vi "Triax320 Init Wait Mess.vi"(7 "Cancelled Ref":refnum<vi>, 8 "error in (no error)":errorcluster, 9 "Stop Ref":refnum<vi>, 10 "Timeout val (ms)":dbl=100.0 min=1.0 step=1.0, 11 "Time Ref":refnum<vi>) -> (0 "error out":errorcluster, 3 "Cancelled Out":bool)   [LabVIEW 2019]
panel:
  out "Progress":u8(slide) scale=0.0..100.0
  out "Time Elapsed":dbl format="%<%M:%S>t"
  in  "stop":bool
  # "Initializing Triax 320 Spectrometer. This may take up to three minutes"
  # "Timeout"
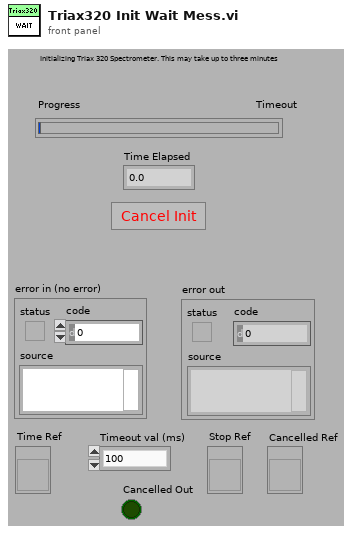
[diagram p1: front panel]
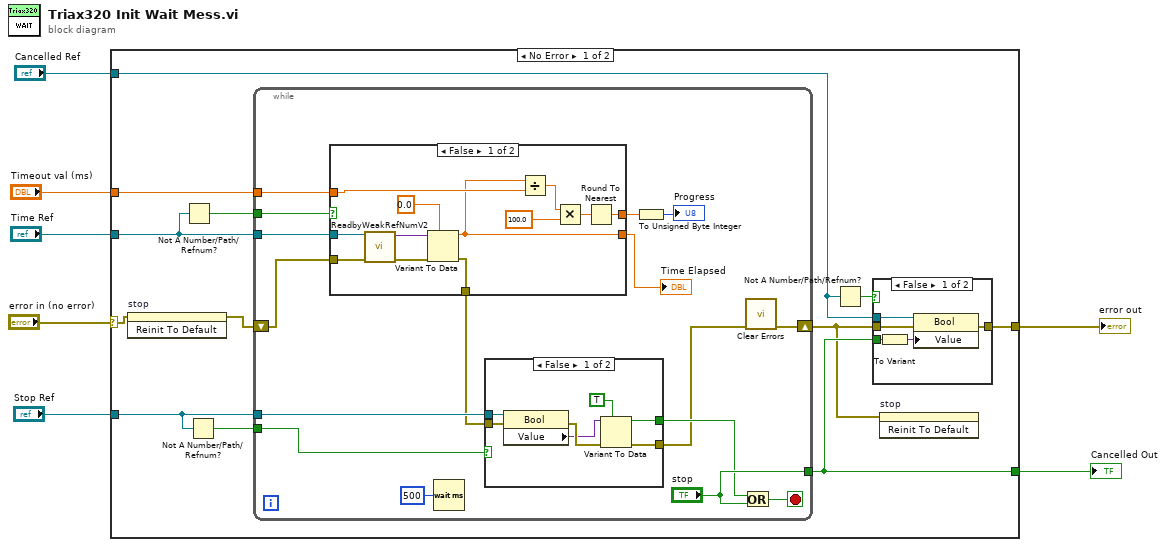
[diagram p0: block diagram]
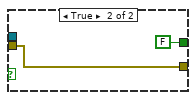
[diagram p3: hidden frame]
diagram:
  n1 = case shown="No Error" "error in (no error)" {
    selector: "error in (no error)" -> [w19 w64]
    tunnel: [w12 w64] -> w6
    tunnel: "Time Ref" -> [w17 _]
    tunnel: "Timeout val (ms)" -> [w15 _]
    tunnel: "Stop Ref" -> [w14 _]
    tunnel: [w11 _] -> w2
    tunnel: "Cancelled Ref" -> [w9 _]
    frame No Error {
      n2 = invoke on="stop" class="Bool (strict)" method="Reinit To Default"(error in=w19) -> (error out=w18:errorcluster)  [unwired: 2 in, 2 out]
      n3 = Not A Number/Path/Refnum?(number/path/refnum=w17) -> (NaN/Path/Refnum?=w16:bool)
      n4 = Not A Number/Path/Refnum?(number/path/refnum=w14) -> (NaN/Path/Refnum?=w13:bool)
      n5 = while {
        shift-right: [w26] -> w8
        shift-left: w18 -> [w38]
        tunnel: w17 -> [w39]
        tunnel: w16 -> [w37]
        tunnel: w15 -> [w36]
        tunnel: w14 -> [w31]
        tunnel: ["stop"] -> w11
        tunnel: w13 -> [w27]
        stop <- w33 stop-if-true
        n6 = case shown="False" w37 {
          tunnel: [w55 _] -> w40
          tunnel: w39 -> [w60 _]
          tunnel: w38 -> [w59 w63]
          tunnel: [w57 w63] -> w28
          tunnel: w36 -> [w56 _]
          tunnel: [w51 _] -> w35
          frame False {
            n7 = call <userlib>:"ReadbyWeakRefNumV2.vi"("error in"=w59, "Control Ref"=w60) -> ("error out"=w58:errorcluster, "Valeur"=w62:variant)  [unwired: 8 in]
            n8 = Variant To Data(error in=w58, type=0.0 ("Time Elapsed"), Variant=w62) -> (data=w55:dbl, error out=w57:errorcluster)
            n9 = Divide(x=w55, y=w56) -> (x/y=w54:dbl)
            n10 = Multiply(x=w54, y=100.0) -> (x*y=w52:dbl)
            n11 = Round To Nearest(number=w52) -> (nearest integer value=w51:dbl)
          }
          frame True {
          }
        }
        "Time Elapsed" <- w40
        n12 = Wait (ms)(milliseconds to wait=u32 500) -> ()  [unwired: 1 out]
        n13 = case shown="False" w27 {
          tunnel: w31 -> [w48 _]
          tunnel: [w44 FALSE ("stop")] -> w30
          tunnel: [w43 w50] -> w29
          tunnel: w28 -> [w42 w50]
          frame False {
            n14 = property class="Bool"(reference=w48, error in=w42) -> (error out=w47:errorcluster, "Value"=w45:variant)  [unwired: 1 out]
            n15 = Variant To Data(error in=w47, type=TRUE ("stop"), Variant=w45) -> (data=w44:bool, error out=w43:errorcluster)
          }
          frame True {
          }
        }
        n16 = To Unsigned Byte Integer(number=w35) -> (unsigned 8bit integer=→"Progress":u8)
        n17 = Or(x=w30, y="stop") -> (x .or. y?=w33:bool)
        n18 = call <vilib>:"Clear Errors.vi"("error in (no error)"=w29) -> ("error out"=w26:errorcluster)  [unwired: 5 in, 1 out]
      }
      n19 = Not A Number/Path/Refnum?(number/path/refnum=w9) -> (NaN/Path/Refnum?=w10:bool)
      n20 = case shown="False" w10 {
        tunnel: w8 -> [w24 w25]
        tunnel: [w23 w25] -> w12
        tunnel: w9 -> [w22 _]
        tunnel: w11 -> [w21 _]
        frame False {
          n21 = To Variant(anything=w21) -> (Variant=w20:variant)
          n22 = property class="Bool"(reference=w22, error in=w24, "Value"=w20) -> (error out=w23:errorcluster)  [unwired: 1 out]
        }
        frame True {
        }
      }
      n23 = invoke on="stop" class="Bool (strict)" method="Reinit To Default"(error in=w8) -> ()  [unwired: 2 in, 3 out]
    }
    frame Error {
    }
  }
  "error out" <- w6
  "Cancelled Out" <- w2
